vi "Action running.vi"() -> ()   [LabVIEW 2023]
panel:
  out "Action running":T1(ring)=enum."pre-reaction"
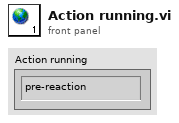
[diagram p1: front panel]
types:
  T1 = enum16{"standby", "pre-reaction", "reaction", "post-reaction", "analysis"}
diagram:
